vi "Kickforce_z.vi"(8 "AI Parameters":T1={"GotoKick"={"Dist do cone a frente"=150.0, "attacker farback"=1500.0, "Perto"=300.0, "min dist to kick"=150.0, "kick eps"=0.05, "Time to transition"=0.0}, "Attacker"={"CC chute"=0.09, "CC passe"=0.045, "Kick Force"=100.0, "ball-robot Kick"=200.0, "ball-robot Pass"=0.3, "drible\nAttk"=FALSE}, "Defender"={"D max"=1700.0, "Vel p/ robô av"=1000.0, "Kick Force"=100.0, "D atk-def"=0.0, "D farback"=0.0, "drible\ndef"=FALSE, "drible\ngoalie"=FALSE}, "Timeout"={"Field/v in x"=6.0, "Dist Robots"=300, "Dist up in y"=300}, "Pose Striker"={"dist"=200.0, "Numeric"=-4.0, "dist 2"=200.0, "drible\nstriker"=FALSE}, "Dist Stop"=300.0, "D ball out"=200, "D central gap "=150.0, "T pass"=0.0, "Force ++"=0.0, "range kick"=0.0, "Chute alto"=TRUE, "Marcador novo"=TRUE, "drible"=FALSE, "D drible"=300.0, "Versão Striker"=enum."Auto", "Defesa"=enum."ManMark", "Marcador"=enum."Marcar Segundo mais perigoso", "Receptor passe"=enum."Auto", "Área"=enum."Quadrada", "Decisão\nsimples?"=FALSE} {"D drible" format="%#_13g"; "D central gap" format="%#_13g"; "Dist Stop" format="%#_13g"; "Pose Striker"."Numeric" format="%#_13g"; "Defender"."Kick Force" format="%#_13g"; "Defender"."Vel p/ robô av" format="%#_13g"; "Attacker"."ball-robot Kick" format="%#_13g"; "Attacker"."Kick Force" format="%#_13g"; "Attacker"."CC passe" format="%#_13g"; "Attacker"."CC chute" format="%#_13g"; "GotoKick"."kick eps" format="%#_13g"; "GotoKick"."min dist to kick" format="%#_13g"; "GotoKick"."Perto" format="%#_13g"; "GotoKick"."attacker farback" format="%#_13g"; "GotoKick"."Dist do cone a frente" format="%#_13g"}, 10 "Distância ao\nalvo do chute":dbl=1.23 format="%#_13g") -> (1 "Tempo até  bola\nchegar ao alvo":dbl, 2 "Força do chute":dbl)   [LabVIEW 2018]
uses:
  AI Parameters.ctl
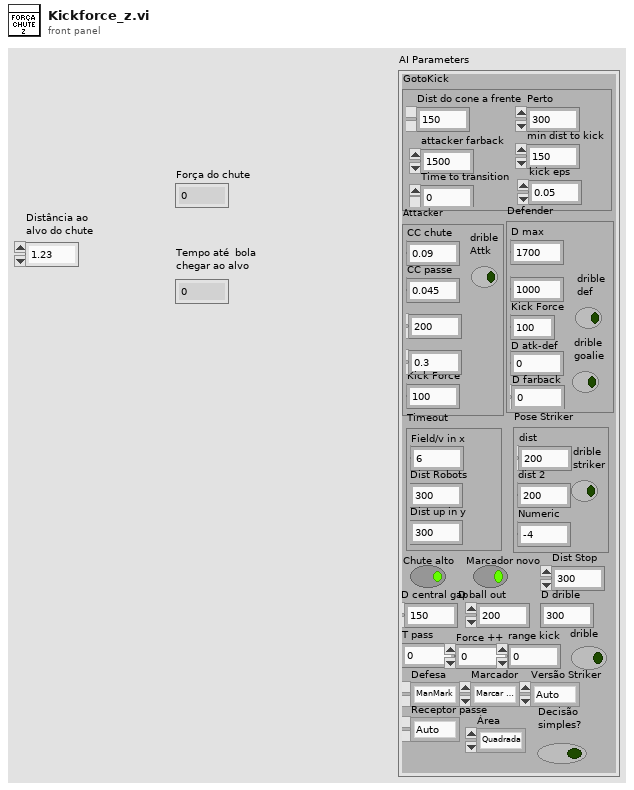
[diagram p1: front panel]
types:
  T1 = typedef "AI Parameters.ctl" = cluster{"GotoKick":cluster{"Dist do cone a frente":dbl, "attacker farback":dbl, "Perto":dbl, "min dist to kick":dbl, "kick eps":dbl, "Time to transition":dbl}, "Attacker":cluster{"CC chute":dbl, "CC passe":dbl, "Kick Force":dbl, "ball-robot Kick":dbl, "ball-robot Pass":dbl, "drible\nAttk":bool}, "Defender":cluster{"D max":dbl, "Vel p/ robô av":dbl, "Kick Force":dbl, "D atk-def":dbl, "D farback":dbl, "drible\ndef":bool, "drible\ngoalie":bool}, "Timeout":cluster{"Field/v in x":dbl, "Dist Robots":u32, "Dist up in y":u32}, "Pose Striker":cluster{"dist":dbl, "Numeric":dbl, "dist 2":dbl, "drible\nstriker":bool}, "Dist Stop":dbl, "D ball out":i32, "D central gap ":dbl, "T pass":dbl, "Force ++":dbl, "range kick":dbl, "Chute alto":bool, "Marcador novo":bool, "drible":bool, "D drible":dbl, "Versão Striker":enum16{"Auto", "3", "2", "1"}, "Defesa":enum16{"ManMark", "Barreira"}, "Marcador":enum16{"Marcar Segundo mais perigoso", "Marcar o mais perigoso"}, "Receptor passe":enum16{"Auto", "2nd Striker", "Striker"}, "Área":enum16{"Quadrada", "Circular"}, "Decisão\nsimples?":bool}
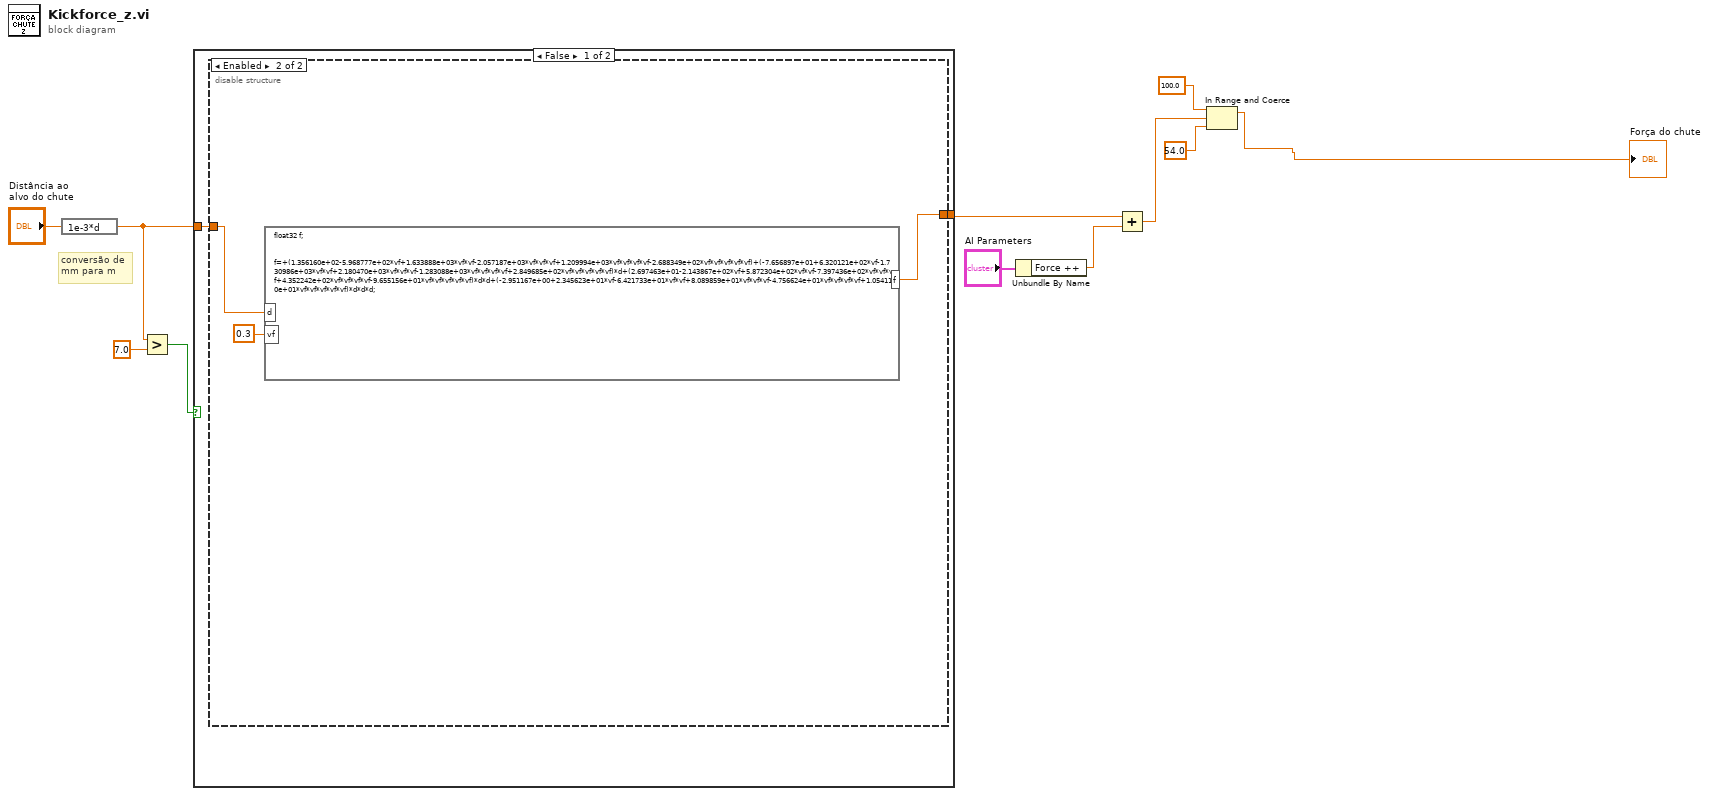
[diagram p0: block diagram]
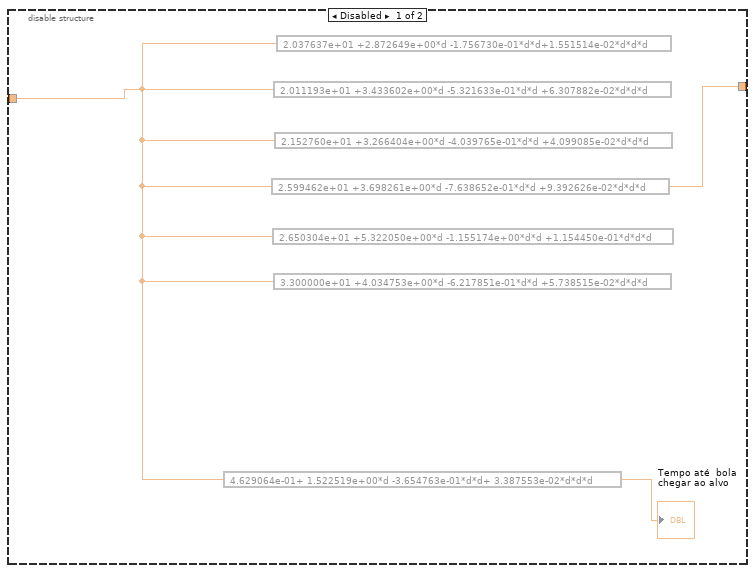
[diagram p2: hidden frame]
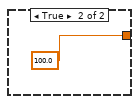
[diagram p3: hidden frame]
diagram:
  # "conversão de\nmm para m"
  n1 = expression code="1e-3*d"("Distância ao\nalvo do chute") -> (w9:dbl)
  n2 = Greater?(x=w9, y=7.0) -> (0:w7:bool)
  n3 = case shown="False" w7 {
    tunnel: w9 -> [w13 _]
    tunnel: [w12 100.0] -> w10
    frame False {
      n4 = disable-structure shown="Enabled" {
        disable-tunnel: w13 -> [w16 w19]
        disable-tunnel: [w14 w18] -> w12
        frame Disabled {
          n5 = expression code="4.629064e-01+ 1.522519e+00*d -3.654763e-01*d*d+ 3.387553e-02*d*d*d"(w16) -> (→"Tempo até  bola\nchegar ao alvo":dbl)
          n6 = expression code="2.599462e+01 +3.698261e+00*d -7.638652e-01*d*d +9.392626e-02*d*d*d"(w16) -> (w14:dbl)
          n7 = expression code="2.650304e+01 +5.322050e+00*d -1.155174e+00*d*d +1.154450e-01*d*d*d"(w16) -> ()  [unwired: 1 out]
          n8 = expression code="2.011193e+01 +3.433602e+00*d -5.321633e-01*d*d +6.307882e-02*d*d*d"(w16) -> ()  [unwired: 1 out]
          n9 = expression code="3.300000e+01 +4.034753e+00*d -6.217851e-01*d*d +5.738515e-02*d*d*d"(w16) -> ()  [unwired: 1 out]
          n10 = expression code="2.152760e+01 +3.266404e+00*d -4.039765e-01*d*d +4.099085e-02*d*d*d"(w16) -> ()  [unwired: 1 out]
          n11 = expression code="2.037637e+01 +2.872649e+00*d -1.756730e-01*d*d+1.551514e-02*d*d*d"(w16) -> ()  [unwired: 1 out]
        }
        frame Enabled {
          n12 = formula code="float32 f;\n\n\nf=+(1.356160e+02-5.968777e+02*vf+1.633888e+03*vf*vf-2.057187e+03*vf*vf*vf+1.209994e+03*vf*vf*vf*vf-2.688349e+02*vf*vf*vf*vf*vf)+(-7.656897e+01+6.320121e+02*vf-1.730986e+03*vf*vf+2.180470e+03*vf*vf*vf-1.283088e+03*vf*vf*vf*vf+2.849685e+02*vf*vf*vf*vf*vf)*d+(2.697463e+01-2.143867e+02*vf+5.872304e+02*vf*vf-7.397436e+02*vf*vf*vf+4.352242e+02*vf*vf*vf*vf-9.655156e+01*vf*vf*vf*vf*vf)*d*d+(-2.951167e+00+2.345623e+01*vf-6.421733e+01*vf*vf+8.089859e+01*vf*vf*vf-4.756624e+01*vf*vf*vf*vf+1.054110e+01*vf*vf*vf*vf*vf)*d*d*d;"("d"=w19, "vf"=0.3 ("input variable")) -> ("f"=w18:sgl)
        }
      }
    }
    frame True {
    }
  }
  n13 = Unbundle By Name("AI Parameters") -> ("Force ++"=w5:dbl)
  n14 = Add(x=w10, y=w5) -> (x+y=w4:dbl)
  n15 = In Range and Coerce(upper limit=100.0, x=w4, lower limit=54.0) -> (coerced(x)=→"Força do chute":dbl)  [unwired: 1 out]
